vi "RGseriesSeria170309.vi"() -> ()   [LabVIEW 2015]
uses:
  <vilib>/Instr/_visa.llb/VISA Configure Serial Port (Instr).vi
  <userlib>/caLab/Private/Put_DBL-1D_PV-1D.vi
  <userlib>/caLab/Private/Get_PV-1D.vi
  <userlib>/caLab/Private/Get_PV.vi
panel:
  in  "PS1:OUT_CNTL":bool
  in  "APX:PS1_V_RV_CNTL":dbl min=0.0 max=5.0 step=0.01
  in  "APX:PS1_I_RV_CNTL":dbl min=0.0 max=0.5 step=0.01
  in  "APX:PS2_V_RV_CNTL":dbl min=0.0 max=3.3 step=0.05
  in  "PS2:OUT_CNTL":bool
  in  "APX:PS2_I_RV_CNTL":dbl min=0.0 max=2.3 step=0.02
  in  "Ring":u16(ring) items=["EPICS", "LOCAL"]
  out "APX:PS2_R_MV":dbl format="%.2f"
  out "APX:PS1_R_MV":dbl format="%.2f"
  out "number 2":dbl
  out "number":dbl
  out "APX:Tpiezo":dbl
  out "APX:Thpc":dbl
  in  "Reset Timer2":bool=TRUE caption="Auto Reset"
  in  "Time Target2 (min)":dbl=1.0 caption="Time Target (s)"
  out "Elapsed Time2 (min)":dbl caption="Elapsed Time (s)"
  out "Time has Elapsed 2":bool caption="Time has Elapsed"
  in  "Timer2":bool
  in  "Timer1":bool
  in  "Reset Timer1":bool=TRUE caption="Auto Reset"
  out "Time has Elapsed":bool
  in  "Time Target1 (min)":dbl=1.0 caption="Time Target (s)"
  out "Elapsed Time (min)":dbl caption="Elapsed Time (s)"
  out "APX:PS1_I_RV":dbl min=0.0 max=0.5 step=0.01
  out "APX:PS1_V_RV":dbl min=0.0 max=5.0 step=0.01
  out "APX:PS1_P_MV":dbl format="%.2f"
  out "APX:PS1_I_MV":dbl format="%.3g"
  out "APX:PS1_V_MV":dbl format="%.3g"
  out "APX:PS1_OUT":bool
  out "APX:Thpc OK?":bool
  out "APX:Tpiezo OK?":bool
  out "APX:PS2_P_MV":dbl format="%.2f"
  out "APX:PS2_I_RV":dbl min=0.0 max=2.3 step=0.02
  out "APX:PS2_OUT":bool
  in  "stop":bool
  out "APX:PS2_I_MV":dbl format="%.3g"
  out "APX:PS2_V_MV":dbl format="%.3g"
  in  "VISA resource name":refnum<visa-resource-name>="COM12"
  out "APX:PS2_V_RV":dbl min=0.0 max=3.3 step=0.05
  # "COM12"
  # "Sample Heater Control"
  # "Cu Mesh Control"
  # "V"
  # "V"
  # "A"
  # "A"
  # "Max 1.2A/0.4x0.1wire"
  # "W"
  # "ohm"
  # "W"
  # "ohm"
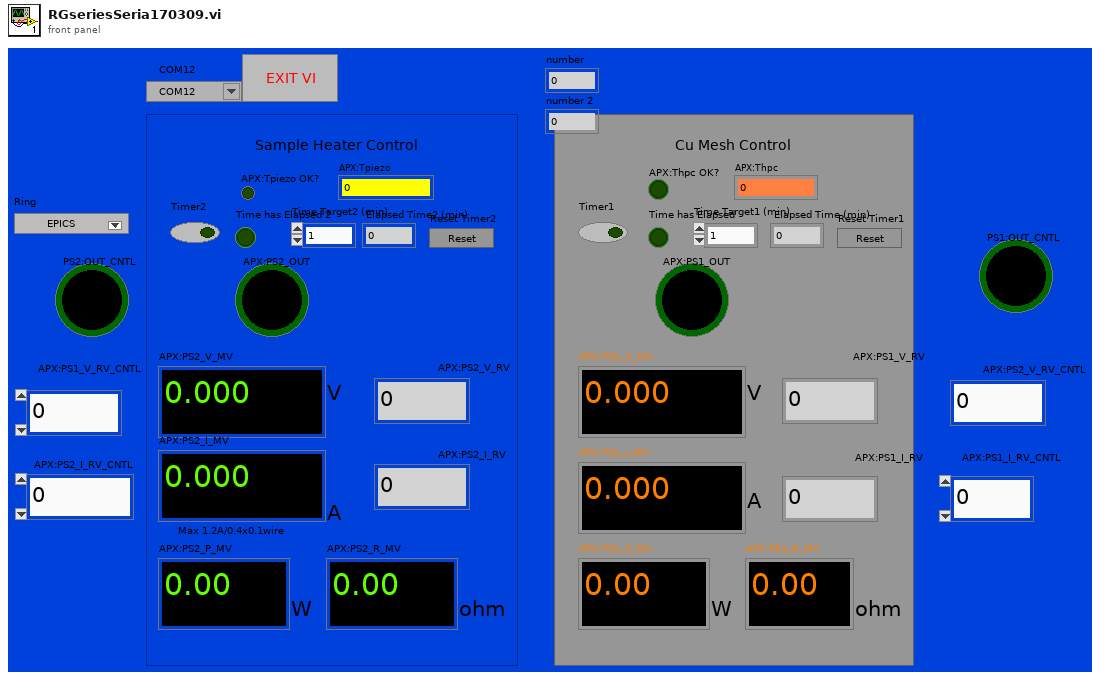
[diagram p1: front panel]
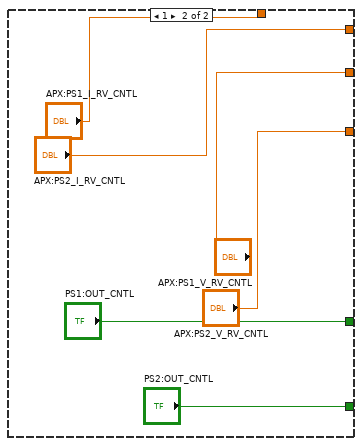
[diagram p2: hidden frame]
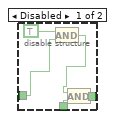
[diagram p4: hidden frame]
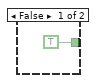
[diagram p6: hidden frame]
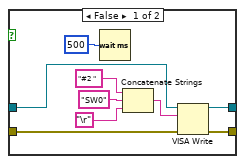
[diagram p8: hidden frame]
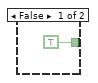
[diagram p11: hidden frame]
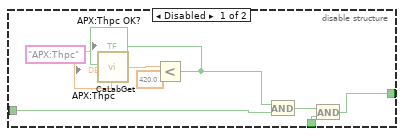
[diagram p13: hidden frame]
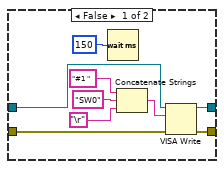
[diagram p14: hidden frame]
diagram:
  # "disable remote control"
  n1 = flat-sequence {
    tunnel: [w50] -> w40
    tunnel: [w49] -> w39
    frame #0 {
      w51 = u16 0 items=["None", "XON/XOFF", "RTS/CTS", "XON/XOFF & RTS/CTS", "DTR/DSR", "XON/XOFF & DTR/DSR"] ("flow control (0:none)")
      w52 = u16 10 items=["1.0"=10, "1.5"=15, "2.0"=20] ("stop bits (10: 1 bit)")
      # "OpenComport"
      # "Stop bits"
      # "enable remote control"
      n2 = call-poly "VISA Configure Serial Port"("VISA resource name"="VISA resource name", "timeout (10sec)"=u32 10000, "baud rate (9600)"=u32 9600, "data bits (8)"=u16 8, "parity (0:none)"=enum16{"None", "Odd", "Even", "Mark", "Space"}."None", "stop bits (10: 1 bit)"=w52, "flow control (0:none)"=w51) -> ("VISA resource name out"=w50:refnum<visa-resource-name>, "error out"=w49:errorcluster)  [unwired: 7 in]
    }
  }
  n3 = flat-sequence {
    tunnel: w40 -> [w63]
    tunnel: w39 -> [w62]
    tunnel: [w59] -> w4
    tunnel: [w58] -> w2
    tunnel: w4 -> [w68]
    tunnel: [w68] -> w3
    tunnel: w2 -> [w67]
    tunnel: [w67] -> w1
    tunnel: [w70] -> w11
    tunnel: [w71] -> w9
    tunnel: w3 -> [w69]
    tunnel: w1 -> [w72]
    frame #0 {
      # "enable output"
      n4 = Concatenate Strings("#2 " ("initial string"), "REN" ("string"), "\r") -> (w64:string)
      n5 = VISA Write(VISA resource name=w63, write buffer=w64, error in (no error)=w62) -> (VISA resource name out=w58:refnum<visa-resource-name>, error out=w59:errorcluster)  [unwired: 1 out]
    }
    frame #1 {
      n6 = Wait (ms)(milliseconds to wait=u32 500) -> ()  [unwired: 1 out]
    }
    frame #2 {
      # "enable output"
      n7 = Concatenate Strings("#1 " ("initial string"), "REN" ("string"), "\r") -> (w76:string)
      n8 = VISA Write(VISA resource name=w72, write buffer=w76, error in (no error)=w69) -> (VISA resource name out=w71:refnum<visa-resource-name>, error out=w70:errorcluster)  [unwired: 1 out]
    }
  }
  n9 = flat-sequence {
    tunnel: w11 -> [w81]
    tunnel: [w81] -> w10
    tunnel: w9 -> [w77]
    tunnel: [w77] -> w8
    tunnel: w10 -> [w92]
    tunnel: w8 -> [w91]
    tunnel: [w92] -> w6
    tunnel: [w91] -> w5
    tunnel: [w94] -> w7
    tunnel: [w95] -> w28
    tunnel: w6 -> [w95]
    tunnel: w5 -> [w94]
    frame #0 {
      n10 = Wait (ms)(milliseconds to wait=u32 500) -> ()  [unwired: 1 out]
      n11 = property on="APX:PS2_I_RV" class="DigNum (strict)"("Value"=0.0 ("APX:RG183_I_RV")) -> ()  [unwired: 2 in, 2 out]
      n12 = property on="APX:PS2_V_RV" class="DigNum (strict)"("Value"=0.0 ("VCN_REQ")) -> ()  [unwired: 2 in, 2 out]
    }
    frame #1 {
      w82 = 0.0 ("VCN_REQ")
      n13 = Build Array("APX:PS1_I_RV" ("format string"), "APX:PS1_V_RV" ("initial string"), "APX:PS2_I_RV" ("format string"), "APX:PS2_V_RV" ("initial string"), "APX:PS1_OUT" ("format string"), "APX:PS2_OUT" ("initial string")) -> (w86:string[])
      n14 = Build Array(w82, w82, w82, w82, w82, w82) -> (w85:dbl[])
      n15 = call-poly "CaLabPut.vi"("Values"=w85, "PV Names"=w86) -> ()  [unwired: 6 in, 4 out]
    }
    frame #2 {
      n16 = Wait (ms)(milliseconds to wait=u32 3000) -> ()  [unwired: 1 out]
    }
  }
  n17 = Concatenate Strings("#2 " ("format string"), "SW0" ("initial string"), "\r" ("input 1")) -> (w42:string)
  n18 = VISA Write(VISA resource name=w7, write buffer=w42, error in (no error)=w28) -> (VISA resource name out=w30:refnum<visa-resource-name>, error out=w29:errorcluster)  [unwired: 1 out]
  n19 = while {
    tunnel: w30 -> [w110]
    tunnel: w29 -> [w111]
    tunnel: [w107] -> w27
    tunnel: [w106] -> w26
    stop <- "stop" stop-if-true
    n20 = case shown="0, Default" "Ring" {
      tunnel: [w122 "APX:PS2_I_RV_CNTL"] -> w103
      tunnel: [w130 "APX:PS1_I_RV_CNTL"] -> w102
      tunnel: [w121 "APX:PS1_V_RV_CNTL"] -> w101
      tunnel: [w113 "PS1:OUT_CNTL"] -> w100
      tunnel: [w112 "PS2:OUT_CNTL"] -> w99
      tunnel: [w120 "APX:PS2_V_RV_CNTL"] -> w98
      frame 0, Default {
        w129 = 0 ("index")
        n21 = Build Array("APX:PS1_I_RV" ("format string"), "APX:PS1_V_RV" ("initial string"), "APX:PS2_I_RV" ("format string"), "APX:PS2_V_RV" ("initial string"), "APX:PS1_OUT" ("format string"), "APX:PS2_OUT" ("initial string")) -> (w133:string[])
        n22 = call-poly <userlib>:"CaLabGet.vi"("PV Names"=w133) -> ("Value Array (number)"=w123:dbl[][])  [unwired: 8 in, 6 out]
        n23 = Index Array(array=w123, index (row)=5, index (col)=w129) -> (element=w118:dbl)
        n24 = Index Array(array=w123, index (row)=4, index (col)=w129) -> (element=w119:dbl)
        n25 = Index Array(array=w123, index (row)=3, index (col)=w129) -> (element=w120:dbl)
        n26 = Index Array(array=w123, index (row)=2, index (col)=w129) -> (element=w121:dbl)
        n27 = Index Array(array=w123, index (row)=0 ("index"), index (col)=0 ("length")) -> (element=w130:dbl)
        n28 = Index Array(array=w123, index (row)=1, index (col)=w129) -> (element=w122:dbl)
        n29 = Number To Boolean Array(number=w119) -> (Boolean array=w117:bool[])
        n30 = Number To Boolean Array(number=w118) -> (Boolean array=w115:bool[])
        n31 = Index Array(array=w117, index=0) -> (element=w113:bool)
        n32 = Index Array(array=w115, index=0) -> (element=w112:bool)
      }
      frame 1 {
      }
    }
    "APX:PS2_V_RV" <- w98
    "APX:PS2_I_RV" <- w103
    "APX:PS2_OUT" <- w99
    "APX:PS1_V_RV" <- w101
    "APX:PS1_I_RV" <- w102
    "APX:PS1_OUT" <- w100
    n33 = flat-sequence {
      tunnel: w111 -> [w164]
      tunnel: w110 -> [w162]
      tunnel: [w166] -> w109
      tunnel: [w165] -> w108
      tunnel: w109 -> [w319]
      tunnel: w108 -> [w318]
      tunnel: [w298] -> w97
      tunnel: [w297] -> w96
      tunnel: [w440] -> w106
      tunnel: [w441] -> w107
      tunnel: w97 -> [w441]
      tunnel: w96 -> [w440]
      frame #0 {
        # "measure current"
        # "measure voltage"
        # "measure voltage"
        # "measure curent"
        # "Measured Voltage"
        # "Measured Current"
        # "Set current"
        # "Set voltage"
        # "disable output"
        n34 = local read "APX:PS2_OUT"() -> (w146:bool)
        n35 = disable-structure shown="Disabled" {
          frame Disabled {
            n36 = call-poly <userlib>:"CaLabGet.vi"("PV Name"="APX:Tpiezo") -> ("1rst Value (number)"=w231:dbl)  [unwired: 8 in, 6 out]
            "APX:Tpiezo" <- w231
            n37 = Less?(x=w231, y=350.0) -> (x < y?=→"APX:Tpiezo OK?":bool)
          }
          frame Enabled {
          }
        }
        n38 = disable-structure shown="Disabled" {
          disable-tunnel: [w239 _] -> w153
          frame Disabled {
            n39 = case shown="True" "Timer2" {
              tunnel: "Time Target2 (min)" -> [_ w246]
              tunnel: [TRUE w245] -> w239
              frame False {
              }
              frame True {
                w250 = 60.0 ("y")
                n40 = Multiply(x=w246, y=w250) -> (x*y=w248:dbl)
                n41 = call "Elapsed Time2"("Time Target (s)"=w248) -> ("Elapsed Time (s)"=w249:dbl, "Time has Elapsed"=w247:bool)  [unwired: 11 in, 6 out]
                "Time has Elapsed 2" <- w247
                n42 = Divide(x=w249, y=w250) -> (x/y=→"Elapsed Time2 (min)":dbl)
                n43 = Not(x=w247) -> (.not. x?=w245:bool)
              }
            }
            n44 = case shown="True" "Reset Timer2" {
              frame False {
              }
              frame True {
                n45 = property on="Elapsed Time2 (min)" class="DigNum (strict)"("Value"=0.0 ("Elapsed Time (min)")) -> ()  [unwired: 2 in, 2 out]
              }
            }
          }
          frame Enabled {
          }
        }
        n46 = disable-structure shown="Enabled" {
          disable-tunnel: w153 -> [w236 _]
          disable-tunnel: [w235 w238] -> w152
          disable-tunnel: w146 -> [w233 w238]
          frame Disabled {
            n47 = And(x=TRUE, y=w233) -> (x .and. y?=w237:bool)
            n48 = And(x=w237, y=w236) -> (x .and. y?=w235:bool)
          }
          frame Enabled {
          }
        }
        n49 = case shown="True" w152 {
          tunnel: w162 -> [w255 w264]
          tunnel: w164 -> [w254 w263]
          tunnel: [w253 w262] -> w163
          tunnel: [w252 w261] -> w161
          frame False {
            n50 = Wait (ms)(milliseconds to wait=u32 500) -> ()  [unwired: 1 out]
            n51 = Concatenate Strings("#2 " ("format string"), "SW0" ("initial string"), "\r" ("input 1")) -> (w257:string)
            n52 = VISA Write(VISA resource name=w255, write buffer=w257, error in (no error)=w254) -> (VISA resource name out=w252:refnum<visa-resource-name>, error out=w253:errorcluster)  [unwired: 1 out]
          }
          frame True {
            n53 = Wait (ms)(milliseconds to wait=u32 150) -> ()  [unwired: 1 out]
            n54 = Concatenate Strings("#2 " ("format string"), "SW1" ("initial string"), "\r" ("input 1")) -> (w266:string)
            n55 = VISA Write(VISA resource name=w264, write buffer=w266, error in (no error)=w263) -> (VISA resource name out=w261:refnum<visa-resource-name>, error out=w262:errorcluster)  [unwired: 1 out]
          }
        }
        n56 = local read "APX:PS2_V_RV"() -> (w148:dbl)
        n57 = In Range and Coerce(upper limit=3.6, x=w148, lower limit=0.0) -> (coerced(x)=w158:dbl)  [unwired: 1 out]
        n58 = flat-sequence {
          tunnel: w161 -> [w282]
          tunnel: w163 -> [w283]
          tunnel: [w283] -> w167
          tunnel: [w282] -> w168
          frame #0 {
            n59 = Wait (ms)(milliseconds to wait=u32 150) -> ()  [unwired: 1 out]
          }
        }
        n60 = Multiply(x=5.5, y=w158) -> (x*y=w226:dbl)
        n61 = Number To Fractional String(number=w226, width (-)=i16 5, precision (6)=i16 2) -> (F-format string=w227:string)  [unwired: 1 in]
        n62 = Concatenate Strings("#2" ("format string"), "VCN " ("initial string"), w227, "\r") -> (w172:string)
        n63 = Concatenate Strings("#2 " ("format string"), "VM" ("initial string"), "\r" ("input 1")) -> (w203:string)
        n64 = VISA Write(VISA resource name=w168, write buffer=w172, error in (no error)=w167) -> (VISA resource name out=w202:refnum<visa-resource-name>, error out=w201:errorcluster)  [unwired: 1 out]
        n65 = VISA Write(VISA resource name=w202, write buffer=w203, error in (no error)=w201) -> (VISA resource name out=w188:refnum<visa-resource-name>, error out=w186:errorcluster)  [unwired: 1 out]
        n66 = local read "APX:PS2_I_RV"() -> (w147:dbl)
        n67 = flat-sequence {
          tunnel: w188 -> [w281]
          tunnel: [w281] -> w187
          tunnel: w186 -> [w280]
          tunnel: [w280] -> w185
          frame #0 {
            n68 = Wait (ms)(milliseconds to wait=u32 150) -> ()  [unwired: 1 out]
          }
        }
        n69 = In Range and Coerce(upper limit=2.8, x=w147, lower limit=0.0) -> (coerced(x)=w155:dbl)  [unwired: 1 out]
        n70 = Multiply(x=33.0, y=w155) -> (x*y=w216:dbl)
        n71 = property class="Instr"(reference=w187, error in=w185) -> (reference out=w194:refnum<visa-resource-name>, error out=w193:errorcluster, "Serial Settings:Number of Bytes at Serial Port"=w192:u32)
        n72 = Number To Fractional String(number=w216, width (-)=i16 5, precision (6)=i16 2) -> (F-format string=w219:string)  [unwired: 1 in]
        n73 = VISA Read(VISA resource name=w194, byte count=w192, error in (no error)=w193) -> (VISA resource name out=w180:refnum<visa-resource-name>, read buffer=w173:string, error out=w179:errorcluster)  [unwired: 1 out]
        n74 = flat-sequence {
          tunnel: w180 -> [w274]
          tunnel: w179 -> [w273]
          tunnel: [w274] -> w177
          tunnel: [w273] -> w178
          frame #0 {
            n75 = Wait (ms)(milliseconds to wait=u32 150) -> ()  [unwired: 1 out]
          }
        }
        n76 = Concatenate Strings("#2 " ("initial string"), "ICN " ("initial string"), w219, "\r") -> (w171:string)
        n77 = String Subset(string=w173, offset (0)=3) -> (substring=w170:string)  [unwired: 1 in]
        n78 = Concatenate Strings("#2 " ("format string"), "IM" ("initial string"), "\r" ("input 1")) -> (w196:string)
        n79 = Fract/Exp String To Number(string=w170) -> (number=w212:dbl)  [unwired: 3 in, 1 out]
        "number 2" <- w212
        n80 = VISA Write(VISA resource name=w177, write buffer=w171, error in (no error)=w178) -> (VISA resource name out=w198:refnum<visa-resource-name>, error out=w199:errorcluster)  [unwired: 1 out]
        n81 = VISA Write(VISA resource name=w198, write buffer=w196, error in (no error)=w199) -> (VISA resource name out=w184:refnum<visa-resource-name>, error out=w183:errorcluster)  [unwired: 1 out]
        n82 = Divide(x=w212, y=5.5 ("x")) -> (x/y=w150:dbl)
        "APX:PS2_V_MV" <- w150
        n83 = flat-sequence {
          tunnel: w184 -> [w277]
          tunnel: w183 -> [w276]
          tunnel: [w277] -> w182
          tunnel: [w276] -> w181
          frame #0 {
            n84 = Wait (ms)(milliseconds to wait=u32 150) -> ()  [unwired: 1 out]
          }
        }
        n85 = property class="Instr"(reference=w182, error in=w181) -> (reference out=w191:refnum<visa-resource-name>, error out=w190:errorcluster, "Serial Settings:Number of Bytes at Serial Port"=w189:u32)
        n86 = VISA Read(VISA resource name=w191, byte count=w189, error in (no error)=w190) -> (VISA resource name out=w176:refnum<visa-resource-name>, read buffer=w174:string, error out=w175:errorcluster)  [unwired: 1 out]
        n87 = flat-sequence {
          tunnel: w176 -> [w271]
          tunnel: w175 -> [w270]
          tunnel: [w271] -> w166
          tunnel: [w270] -> w165
          frame #0 {
            n88 = Wait (ms)(milliseconds to wait=u32 150) -> ()  [unwired: 1 out]
          }
        }
        n89 = String Subset(string=w174, offset (0)=3) -> (substring=w169:string)  [unwired: 1 in]
        n90 = Fract/Exp String To Number(string=w169) -> (number=w209:dbl)  [unwired: 3 in, 1 out]
        "number" <- w209
        n91 = Divide(x=w209, y=33.5 ("x")) -> (x/y=w151:dbl)
        "APX:PS2_I_MV" <- w151
        n92 = Divide(x=w150, y=w151) -> (x/y=→"APX:PS2_R_MV":dbl)
        n93 = Multiply(x=w150, y=w151) -> (x*y=→"APX:PS2_P_MV":dbl)
      }
      frame #1 {
        # "measure curent"
        # "Measured Voltage"
        # "Measured Current"
        # "disable output"
        # "measure current"
        # "measure voltage"
        # "Set current"
        # "measure voltage"
        # "Set voltage"
        n94 = disable-structure shown="Disabled" {
          disable-tunnel: [w369 _] -> w291
          frame Disabled {
            n95 = case shown="True" "Timer1" {
              tunnel: "Time Target1 (min)" -> [_ w374]
              tunnel: [TRUE w373] -> w369
              frame False {
              }
              frame True {
                w378 = 60.0 ("y")
                n96 = Multiply(x=w374, y=w378) -> (x*y=w376:dbl)
                n97 = call "Elapsed Time"("Time Target (s)"=w376) -> ("Elapsed Time (s)"=w377:dbl, "Time has Elapsed"=w375:bool)  [unwired: 11 in, 6 out]
                "Time has Elapsed" <- w375
                n98 = Divide(x=w377, y=w378) -> (x/y=→"Elapsed Time (min)":dbl)
                n99 = Not(x=w375) -> (.not. x?=w373:bool)
              }
            }
          }
          frame Enabled {
          }
        }
        n100 = local read "APX:PS1_OUT"() -> (w285:bool)
        n101 = disable-structure shown="Enabled" {
          disable-tunnel: w285 -> [w383 w388]
          disable-tunnel: [w381 w388] -> w292
          disable-tunnel: w291 -> [w380 _]
          frame Disabled {
            n102 = call-poly <userlib>:"CaLabGet.vi"("PV Name"="APX:Thpc") -> ("1rst Value (number)"=w386:dbl)  [unwired: 8 in, 6 out]
            "APX:Thpc" <- w386
            n103 = Less?(x=w386, y=420.0) -> (x < y?=w384:bool)
            "APX:Thpc OK?" <- w384
            n104 = And(x=w384, y=w383) -> (x .and. y?=w382:bool)
            n105 = And(x=w382, y=w380) -> (x .and. y?=w381:bool)
          }
          frame Enabled {
          }
        }
        n106 = disable-structure shown="Disabled" {
          frame Disabled {
            n107 = case shown="True" "Reset Timer1" {
              frame False {
              }
              frame True {
                n108 = property on="Elapsed Time (min)" class="DigNum (strict)"("Value"=0.0 ("Elapsed Time (min)")) -> ()  [unwired: 2 in, 2 out]
              }
            }
          }
          frame Enabled {
          }
        }
        n109 = local read "APX:PS1_V_RV"() -> (w287:dbl)
        n110 = case shown="True" w292 {
          tunnel: w319 -> [w401 w410]
          tunnel: w318 -> [w400 w409]
          tunnel: [w399 w408] -> w317
          tunnel: [w398 w407] -> w316
          frame False {
            n111 = Wait (ms)(milliseconds to wait=u32 150) -> ()  [unwired: 1 out]
            n112 = Concatenate Strings("#1 " ("format string"), "SW0" ("initial string"), "\r" ("input 1")) -> (w405:string)
            n113 = VISA Write(VISA resource name=w401, write buffer=w405, error in (no error)=w400) -> (VISA resource name out=w398:refnum<visa-resource-name>, error out=w399:errorcluster)  [unwired: 1 out]
          }
          frame True {
            n114 = Wait (ms)(milliseconds to wait=u32 150) -> ()  [unwired: 1 out]
            n115 = Concatenate Strings("#1 " ("format string"), "SW1" ("initial string"), "\r" ("input 1")) -> (w414:string)
            n116 = VISA Write(VISA resource name=w410, write buffer=w414, error in (no error)=w409) -> (VISA resource name out=w407:refnum<visa-resource-name>, error out=w408:errorcluster)  [unwired: 1 out]
          }
        }
        n117 = In Range and Coerce(upper limit=5.01, x=w287, lower limit=0.0) -> (coerced(x)=w330:dbl)  [unwired: 1 out]
        n118 = flat-sequence {
          tunnel: [w417] -> w314
          tunnel: w317 -> [w417]
          tunnel: [w416] -> w315
          tunnel: w316 -> [w416]
          frame #0 {
            n119 = Wait (ms)(milliseconds to wait=u32 150) -> ()  [unwired: 1 out]
          }
        }
        n120 = Multiply(x=5.55, y=w330) -> (x*y=w322:dbl)
        n121 = Number To Fractional String(number=w322, width (-)=i16 5, precision (6)=i16 2) -> (F-format string=w321:string)  [unwired: 1 in]
        n122 = Concatenate Strings("#1" ("format string"), "VCN " ("initial string"), w321, "\r") -> (w335:string)
        n123 = Concatenate Strings("#1" ("format string"), "VM" ("initial string"), "\r" ("input 1")) -> (w334:string)
        n124 = VISA Write(VISA resource name=w315, write buffer=w335, error in (no error)=w314) -> (VISA resource name out=w336:refnum<visa-resource-name>, error out=w362:errorcluster)  [unwired: 1 out]
        n125 = VISA Write(VISA resource name=w336, write buffer=w334, error in (no error)=w362) -> (VISA resource name out=w363:refnum<visa-resource-name>, error out=w364:errorcluster)  [unwired: 1 out]
        n126 = flat-sequence {
          tunnel: w363 -> [w421]
          tunnel: [w421] -> w365
          tunnel: w364 -> [w420]
          tunnel: [w420] -> w366
          frame #0 {
            n127 = Wait (ms)(milliseconds to wait=u32 150) -> ()  [unwired: 1 out]
          }
        }
        n128 = property class="Instr"(reference=w365, error in=w366) -> (reference out=w358:refnum<visa-resource-name>, error out=w359:errorcluster, "Serial Settings:Number of Bytes at Serial Port"=w360:u32)
        n129 = local read "APX:PS1_I_RV"() -> (w286:dbl)
        n130 = VISA Read(VISA resource name=w358, byte count=w360, error in (no error)=w359) -> (VISA resource name out=w296:refnum<visa-resource-name>, read buffer=w361:string, error out=w294:errorcluster)  [unwired: 1 out]
        n131 = String Subset(string=w361, offset (0)=3) -> (substring=w351:string)  [unwired: 1 in]
        n132 = flat-sequence {
          tunnel: w296 -> [w391]
          tunnel: [w391] -> w295
          tunnel: [w389] -> w293
          tunnel: w294 -> [w389]
          frame #0 {
            n133 = Wait (ms)(milliseconds to wait=u32 150) -> ()  [unwired: 1 out]
          }
        }
        n134 = In Range and Coerce(upper limit=0.501, x=w286, lower limit=0.0) -> (coerced(x)=w354:dbl)  [unwired: 1 out]
        n135 = Fract/Exp String To Number(string=w351) -> (number=w345:dbl)  [unwired: 3 in, 1 out]
        n136 = Divide(x=w345, y=5.55 ("x")) -> (x/y=w290:dbl)
        "APX:PS1_V_MV" <- w290
        n137 = Multiply(x=37.35, y=w354) -> (x*y=w341:dbl)
        n138 = Number To Fractional String(number=w341, width (-)=i16 5, precision (6)=i16 2) -> (F-format string=w338:string)  [unwired: 1 in]
        n139 = Concatenate Strings("#1 " ("initial string"), "ICN " ("initial string"), w338, "\r") -> (w355:string)
        n140 = Concatenate Strings("#1 " ("format string"), "IM" ("initial string"), "\r" ("input 1")) -> (w356:string)
        n141 = VISA Write(VISA resource name=w295, write buffer=w355, error in (no error)=w293) -> (VISA resource name out=w357:refnum<visa-resource-name>)  [unwired: 2 out]
        n142 = VISA Write(VISA resource name=w357, write buffer=w356) -> (VISA resource name out=w301:refnum<visa-resource-name>, error out=w300:errorcluster)  [unwired: 1 in, 1 out]
        n143 = flat-sequence {
          tunnel: w301 -> [w396]
          tunnel: w300 -> [w395]
          tunnel: [w396] -> w307
          tunnel: [w395] -> w306
          frame #0 {
            n144 = Wait (ms)(milliseconds to wait=u32 150) -> ()  [unwired: 1 out]
          }
        }
        n145 = property class="Instr"(reference=w307, error in=w306) -> (reference out=w310:refnum<visa-resource-name>, error out=w309:errorcluster, "Serial Settings:Number of Bytes at Serial Port"=w308:u32)
        n146 = VISA Read(VISA resource name=w310, byte count=w308, error in (no error)=w309) -> (VISA resource name out=w305:refnum<visa-resource-name>, read buffer=w303:string, error out=w304:errorcluster)  [unwired: 1 out]
        n147 = String Subset(string=w303, offset (0)=3) -> (substring=w302:string)  [unwired: 1 in]
        n148 = flat-sequence {
          tunnel: w305 -> [w393]
          tunnel: w304 -> [w392]
          tunnel: [w393] -> w298
          tunnel: [w392] -> w297
          frame #0 {
            n149 = Wait (ms)(milliseconds to wait=u32 150) -> ()  [unwired: 1 out]
          }
        }
        n150 = Fract/Exp String To Number(string=w302) -> (number=w312:dbl)  [unwired: 3 in, 1 out]
        n151 = Divide(x=w312, y=33.3 ("x")) -> (x/y=w289:dbl)
        "APX:PS1_I_MV" <- w289
        n152 = Divide(x=w290, y=w289) -> (x/y=→"APX:PS1_R_MV":dbl)
        n153 = Multiply(x=w290, y=w289) -> (x*y=→"APX:PS1_P_MV":dbl)
      }
      frame #2 {
        n154 = local read "APX:PS2_I_MV"() -> (w428:dbl)
        n155 = local read "APX:PS1_V_MV"() -> (w427:dbl)
        n156 = local read "APX:PS1_I_MV"() -> (w429:dbl)
        n157 = local read "APX:PS2_P_MV"() -> (w422:dbl)
        n158 = local read "APX:PS2_R_MV"() -> (w424:dbl)
        n159 = local read "APX:PS2_V_MV"() -> (w426:dbl)
        n160 = local read "APX:PS1_R_MV"() -> (w425:dbl)
        n161 = local read "APX:PS1_P_MV"() -> (w423:dbl)
        n162 = Build Array("APX:PS1_I_MV" ("format string"), "APX:PS2_/i_MV" ("initial string"), "APX:PS1_V_MV" ("format string"), "APX:PS2_V_MV" ("initial string"), "APX:PS1_R_MV" ("format string"), "APX:PS2_R_MV" ("initial string"), "APX:PS1_P_MV" ("format string"), "APX:PS2_P_MV" ("initial string")) -> (w435:string[])
        n163 = Build Array(w429, w428, w427, w426, w425, w424, w423, w422) -> (w434:dbl[])
        n164 = call-poly "CaLabPut.vi"("Values"=w434, "PV Names"=w435) -> ()  [unwired: 6 in, 4 out]
      }
    }
  }
  n165 = Concatenate Strings("#2 " ("format string"), "SW0" ("initial string"), "\r" ("input 1")) -> (w36:string)
  n166 = VISA Write(VISA resource name=w27, write buffer=w36, error in (no error)=w26) -> (VISA resource name out=w32:refnum<visa-resource-name>, error out=w31:errorcluster)  [unwired: 1 out]
  n167 = Concatenate Strings("#2 " ("initial string"), "\r", "GTL" ("input 1")) -> (w41:string)
  n168 = VISA Write(VISA resource name=w32, write buffer=w41, error in (no error)=w31) -> (VISA resource name out=w15:refnum<visa-resource-name>, error out=w14:errorcluster)  [unwired: 1 out]
  n169 = Concatenate Strings("#1 " ("format string"), "SW0" ("initial string"), "\r" ("input 1")) -> (w21:string)
  n170 = VISA Write(VISA resource name=w15, write buffer=w21, error in (no error)=w14) -> (VISA resource name out=w17:refnum<visa-resource-name>, error out=w16:errorcluster)  [unwired: 1 out]
  n171 = Concatenate Strings("#1" ("initial string"), "\r", "GTL" ("input 1")) -> (w22:string)
  n172 = VISA Write(VISA resource name=w17, write buffer=w22, error in (no error)=w16) -> (VISA resource name out=w13:refnum<visa-resource-name>, error out=w12:errorcluster)  [unwired: 1 out]
  n173 = flat-sequence {
    tunnel: w13 -> [w446]
    tunnel: w12 -> [w445]
    tunnel: [w446] -> w38
    tunnel: [w445] -> w37
    frame #0 {
      n174 = Wait (ms)(milliseconds to wait=u32 100) -> ()  [unwired: 1 out]
      n175 = property on="APX:PS2_OUT" class="Bool (strict)"("Value"=FALSE ("Output")) -> ()  [unwired: 2 in, 2 out]
      n176 = property on="APX:PS2_V_RV" class="DigNum (strict)"("Value"=0.0 ("VCN_REQ")) -> ()  [unwired: 2 in, 2 out]
      n177 = property on="APX:PS2_I_RV" class="DigNum (strict)"("Value"=0.0 ("APX:RG183_I_RV")) -> ()  [unwired: 2 in, 2 out]
    }
  }
  n178 = VISA Close(VISA resource name=w38, error in (no error)=w37) -> ()  [unwired: 1 out]
